vi "Executable Set Version__icon_lib_labview_project_api.vi"(8 "error in (no error)":errorcluster, 10 "Version":T1, 11 "Build Spec Reference":refnum<vi>) -> (0 "error out":errorcluster, 3 "Build Spec Reference Dup":refnum<vi>)   [LabVIEW 2016, in "LabVIEW Project API__icon_lib_labview_project_api.lvlib"]
doc: "Returns a Build Specification Executable Version [Major, Minor, Fix, Build]\n\n<b>Author:</b> JG\n\n<b>ICON Technologies Pty Ltd</b>\nCopyright (C) 1990-2009\nAll Rights Reserved"
uses:
  LabVIEW Project API__icon_lib_labview_project_api.lvlib
panel:
  # "Output"
  # "Input"
  # "ICON Technologies Pty Ltd\nCopyright (C) 1990-2009\nAll Rights Reserved"
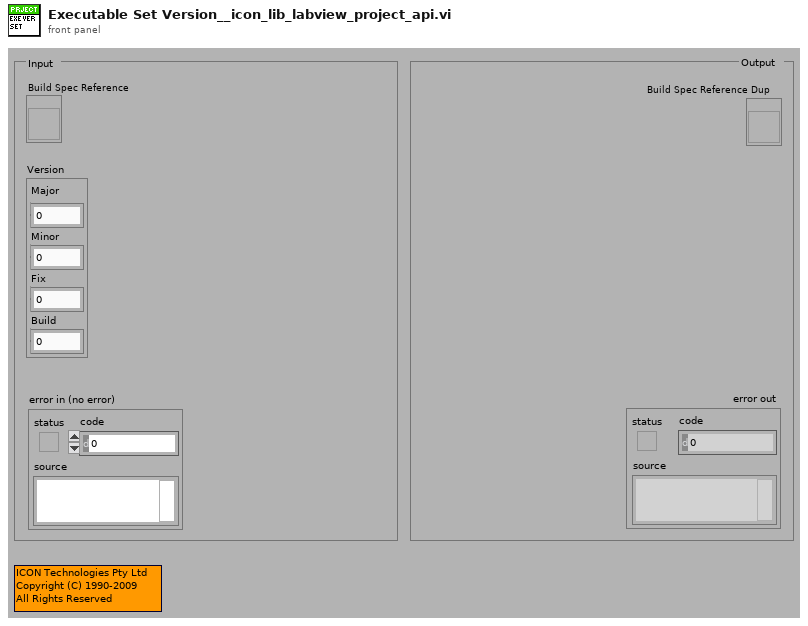
[diagram p1: front panel]
types:
  T1 = cluster{"Major":u16, "Minor":u16, "Fix":u16, "Build":u16}
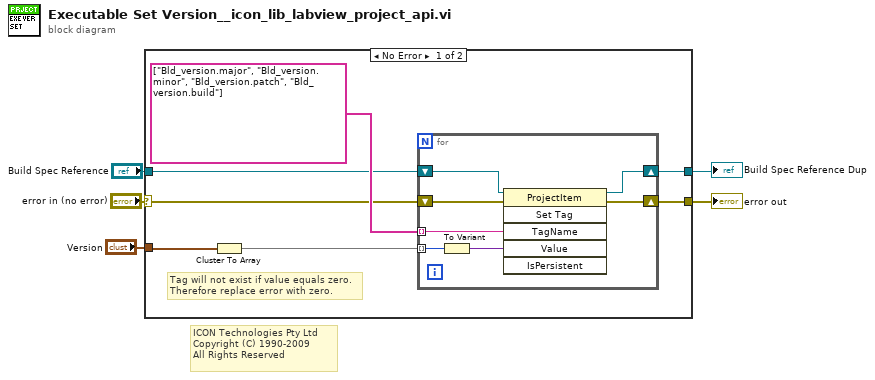
[diagram p0: block diagram]
diagram:
  # "ICON Technologies Pty Ltd\nCopyright (C) 1990-2009\nAll Rights Reserved"
  n1 = case shown="No Error" "error in (no error)" {
    selector: "error in (no error)" -> [w9 w21]
    tunnel: [w11 w21] -> w4
    tunnel: "Build Spec Reference" -> [w10 w20]
    tunnel: [w8 w20] -> w2
    tunnel: "Version" -> [w7 _]
    frame No Error {
      # "Tag will not exist if value equals zero.\nTherefore replace error with zero."
      n2 = Cluster To Array(cluster=w7) -> (array=w6:u16[])
      n3 = for {
        shift-right: [w17] -> w8
        shift-left: w10 -> [w19]
        shift-right: [w13] -> w11
        shift-left: w9 -> [w18]
        tunnel: string[] ["Bld_version.major", "Bld_version.minor", "Bld_version.patch", "Bld_version.build"] -> [w16] mode=indexing
        tunnel: w6 -> [w15] mode=indexing
        n4 = To Variant(anything=w15) -> (Variant=w14:variant)
        n5 = invoke class="ProjectItem" method="Set Tag"(reference=w19, error in=w18, "TagName"=w16, "Value"=w14) -> (reference out=w17:refnum<vi>, error out=w13:errorcluster)  [unwired: 2 in, 4 out]
      }
    }
    frame Error {
    }
  }
  "error out" <- w4
  "Build Spec Reference Dup" <- w2
